vi "Move Pen.vi"(3 "absolute coordinates?(T)":bool=TRUE, 4 "new position":cluster{"x":i16, "y":i16}, 5 "picture":picture) -> (2 "new picture":picture)   [LabVIEW 2020]
doc: "Changes the current pen location of a picture to the specified position or by the specified amount if the position is relative."
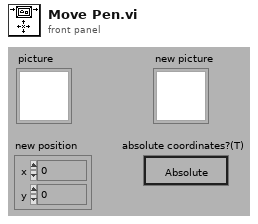
[diagram p1: front panel]
types:
  T1 = cluster{"opcode-Move":i16, "size":i32, cluster{"y":i16, "x":i16}}
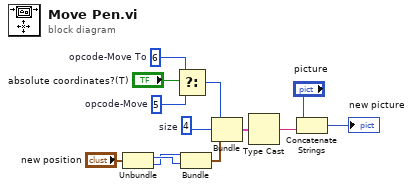
[diagram p0: block diagram]
diagram:
  w11 = i16 5  # opcode-Move
  w12 = i16 6  # opcode-Move To
  w8 = 4  # size
  n1 = Unbundle("new position") -> ("x"=w2:i16, "y"=w1:i16)
  n2 = Select(t=w12, s="absolute coordinates?(T)", f=w11) -> (s? t:f=w10:i16)
  n3 = Bundle("y"=w1, "x"=w2) -> (w3:cluster{"y":i16, "x":i16})  [unwired: 1 in]
  n4 = Bundle("opcode-Move"=w10, "size"=w8, w3) -> (w9:T1)  [unwired: 1 in]
  n5 = Type Cast(x=w9) -> (*(type *) &x=w6:string)  [unwired: 1 in]
  n6 = Concatenate Strings("picture", w6) -> (→"new picture":picture)
